vi "RouteExternalInterfaces.vi"(7 "ObjectName":string, 8 "error in (no error)":errorcluster, 9 "ConfigObject":refnum<class "IApplicationConfiguration.lvclass">, 10 "ITAFObject in":refnum<class "ITAFObject.lvclass">, 11 "Variant in":variant) -> (0 "error out":errorcluster, 3 "Variant out":variant)   [LabVIEW 2021, in "Application.lvclass"]
uses:
  Application.lvclass
  Interface_TAF_IApplicationConfiguration/IApplicationConfiguration/IApplicationConfiguration.lvclass
  Interface_TAF_ITAFObject/ITAFObject/ITAFObject.lvclass
  IInterface/IInterface.lvclass
  c3e78f46-7d6b-47a7-82af-8d499459744c.vi
  <vilib>/TriekselSoft/TracerLibrary/TracerLibrary/Tracer/protected/SendMessage.vi
  <vilib>/TriekselSoft/TracerLibrary/TracerLibrary/Tracer/protected/Timestamp.vi
  c3e78f46-7d6b-47a7-82af-8d499459744c.vi/f75db090-0877-4668-94fb-75c2140b1617.vi
  <vilib>/TriekselSoft/TracerLibrary/TracerLibrary/Tracer/Tracer_Level-Debug.vi
  <vilib>/JDP Science/JSONtext/Variant to JSON Text.vi
  <vilib>/TriekselSoft/TracerLibrary/TracerLibrary/Tracer/protected/Tracer_ClassAttributes.vi
  <vilib>/JDP Science/JSONtext/LVClass Serializer/JSONtext LVClass Serializer.lvclass
  Application.lvclass/Application.ctl
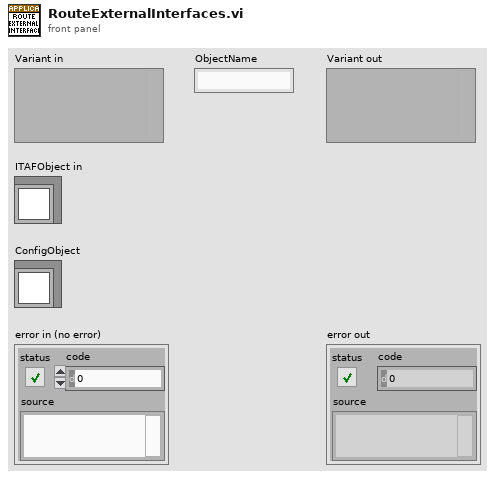
[diagram p1: front panel]
types:
  T1 = typedef "ClusterArrayConversion.lvlib/BundledArray.ctl" = cluster{"Label":string, "Object":refnum<class>, "Array":bool}
  T2 = cluster{"ObjectName":string, "Label":string, "error out":errorcluster}
  T3 = cluster{"ObjectName":string, "Label":string, "ClassName":string}
  T4 = cluster{"ObjectName":string, "Label":string, "class name":string}
  T5 = typedef "IApplicationConfiguration.lvclass/ObjectData.ctl" = cluster{"Label":string, "ObjectName":string, "Type":string}
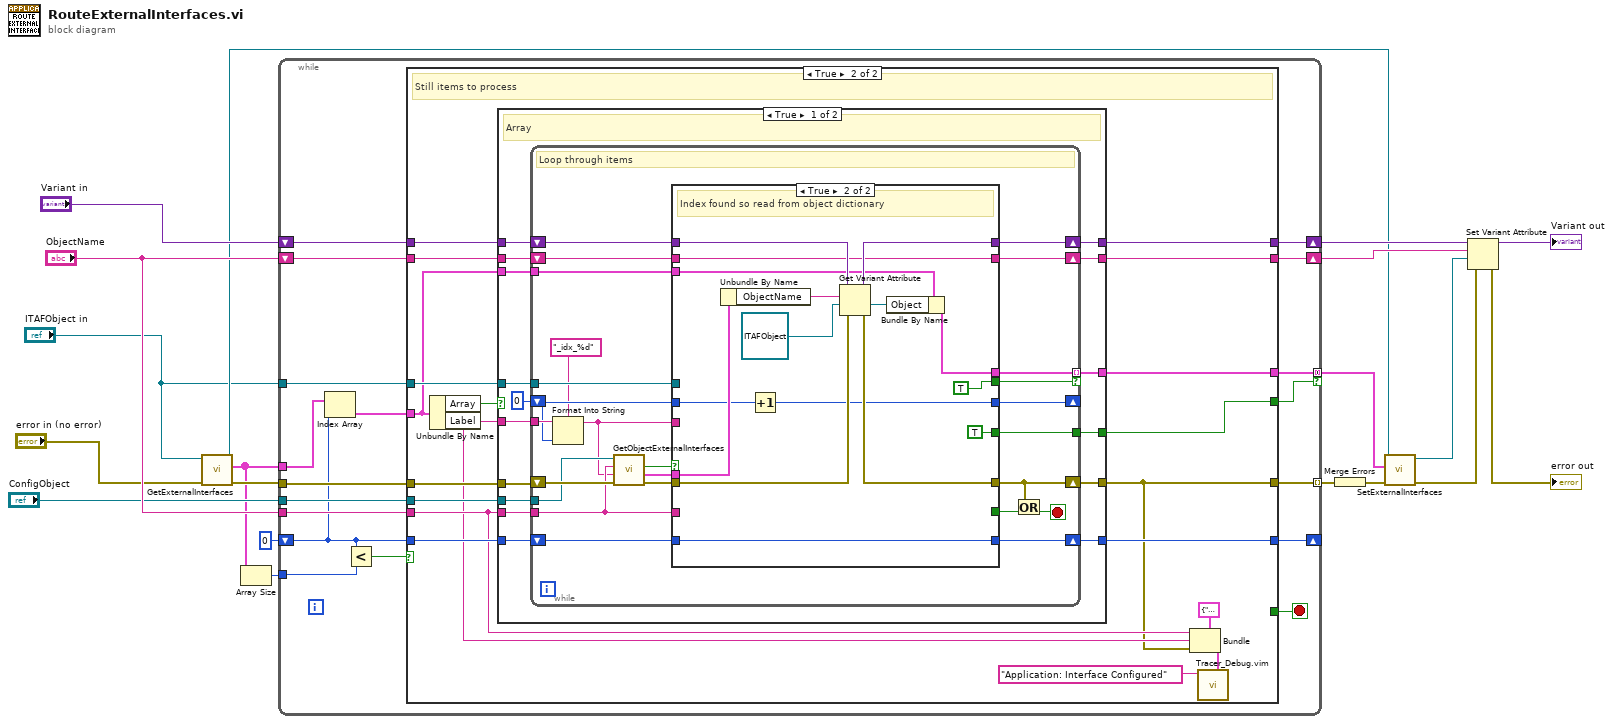
[diagram p0: block diagram]
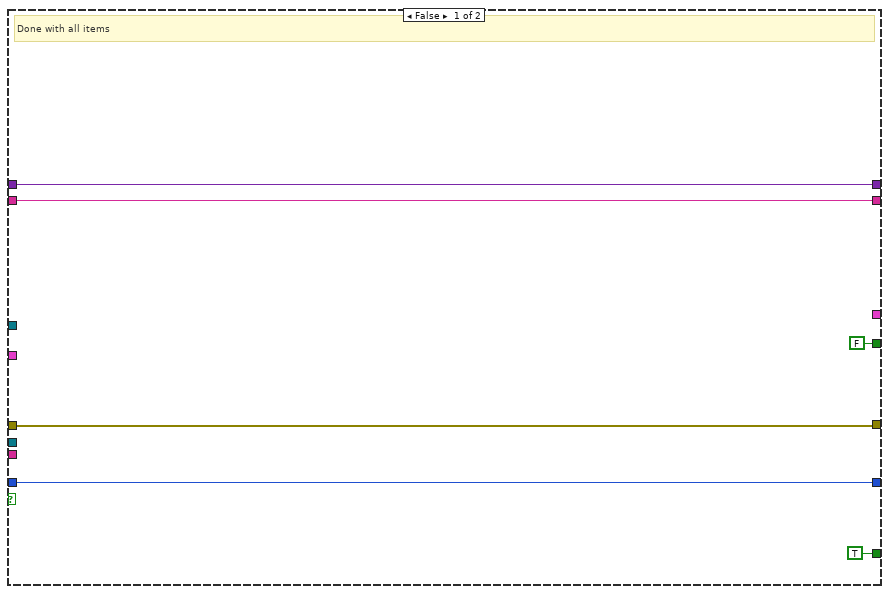
[diagram p2: hidden frame]
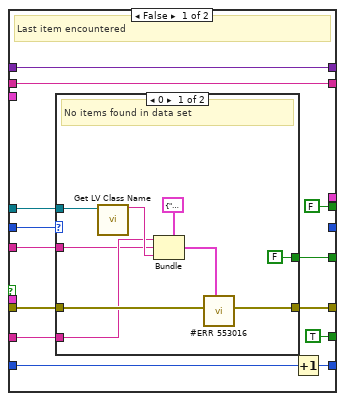
[diagram p3: hidden frame]
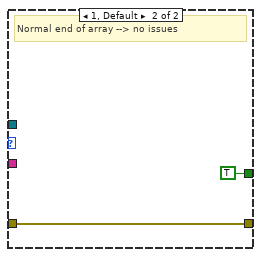
[diagram p4: hidden frame]
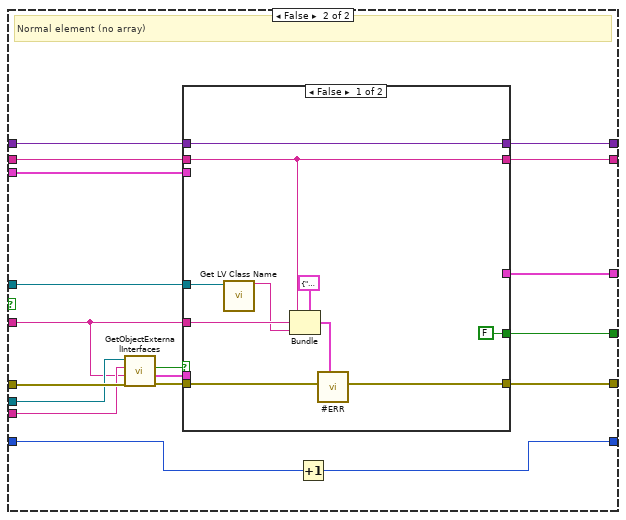
[diagram p5: hidden frame]
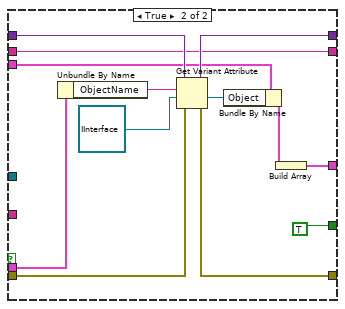
[diagram p6: hidden frame]
diagram:
  n1 = call-dynamic "GetExternalInterfaces.vi"("Error In"="error in (no error)", "object in"="ITAFObject in") -> ("Error Out"=w8:errorcluster, "ExternalInterfaces"=w4:T1[], "object out"=w10:refnum<class "ITAFObject.lvclass">)  [unwired: 7 in]
  n2 = Array Size(array=w4) -> (size(s)=w3:i32)
  n3 = while {
    tunnel: [w37] -> w9 mode=concatenating if=w22
    shift-right: [w33] -> w14
    shift-left: "Variant in" -> [w36]
    shift-right: [w31] -> w15
    shift-left: "ObjectName" -> [w32]
    tunnel: "ConfigObject" -> [w34]
    tunnel: "ObjectName" -> [w30]
    tunnel: w8 -> [w35]
    tunnel: [w29] -> w19 mode=indexing
    tunnel: "ITAFObject in" -> [w28]
    shift-right: [w26] -> _
    shift-left: 0 -> [w25]
    tunnel: w3 -> [w24]
    tunnel: w4 -> [w21]
    stop <- w20 stop-if-true
    n4 = Index Array(array=w21, index=w25) -> (element=w27:T1)
    n5 = Less?(x=w25, y=w24) -> (x < y?=w23:bool)
    n6 = case shown="True" w23 {
      tunnel: [_ w62] -> w37
      tunnel: w36 -> [w43 w61]
      tunnel: w35 -> [w40 w60]
      tunnel: w34 -> [_ w59]
      tunnel: [w43 w58] -> w33
      tunnel: w32 -> [w42 w57]
      tunnel: [w42 w56] -> w31
      tunnel: w30 -> [_ w48]
      tunnel: [w40 w46] -> w29
      tunnel: w28 -> [_ w55]
      tunnel: w27 -> [_ w44]
      tunnel: [w39 w54] -> w26
      tunnel: w25 -> [w39 w53]
      tunnel: [FALSE w45] -> w22
      tunnel: [TRUE _] -> w20
      frame False {
        # "Done with all items"
      }
      frame True {
        # "Still items to process"
        n7 = Unbundle By Name(w44) -> ("Array"=w52:bool, "Label"=w47:string)
        n8 = case shown="True" w52 {
          tunnel: [w78 w161] -> w62
          tunnel: w61 -> [w77 w160]
          tunnel: w60 -> [w76 w159]
          tunnel: w59 -> [w75 w158]
          tunnel: [w74 w155] -> w58
          tunnel: w57 -> [w73 w153]
          tunnel: [w72 w152] -> w56
          tunnel: w48 -> [w71 w151]
          tunnel: [w65 w150] -> w46
          tunnel: w47 -> [w70 w149]
          tunnel: w55 -> [w69 w148]
          tunnel: [w68 w146] -> w54
          tunnel: w53 -> [w67 w147]
          tunnel: [w64 w145] -> w45
          tunnel: w44 -> [w63 w144]
          frame True {
            # "Array"
            n9 = while {
              tunnel: w75 -> [w100]
              tunnel: w71 -> [w84]
              tunnel: w70 -> [w90]
              tunnel: w69 -> [w93]
              shift-right: [w97] -> w74
              shift-left: w77 -> [w102]
              shift-right: [w81] -> w65
              shift-left: w76 -> [w101]
              shift-right: [w94] -> w72
              shift-left: w73 -> [w95]
              shift-right: [w92] -> w68
              shift-left: w67 -> [w91]
              shift-right: [w87] -> _
              shift-left: 0 -> [w89]
              tunnel: [w103] -> w78 mode=indexing if=w86
              tunnel: [w80] -> w64
              tunnel: w63 -> [w79]
              stop <- w82 stop-if-true
              # "Loop through items"
              n10 = Format Into String(format string="_idx_%d", initial string=w90, w89) -> (resulting string=w83:string)  [unwired: 1 in, 1 out]
              n11 = call-dynamic "GetObjectExternalInterfaces.vi"("Error In"=w101, "Label"=w83, "ThisObject"=w84, "object in"=w100) -> ("Error Out"=w98:errorcluster, "ObjectData"=w99:T5, "Valid"=w96:bool)  [unwired: 4 in, 1 out]
              n12 = case shown="True" w96 {
                tunnel: [_ w143] -> w103
                tunnel: w102 -> [w113 w142]
                tunnel: w99 -> [_ w141]
                tunnel: w98 -> [w116 w138]
                tunnel: [w115 w137] -> w81
                tunnel: [w113 w136] -> w97
                tunnel: w84 -> [w114 _]
                tunnel: [w112 w134] -> w94
                tunnel: w95 -> [w112 w134]
                tunnel: w83 -> [w111 _]
                tunnel: w93 -> [w110 _]
                tunnel: w91 -> [w106 w133]
                tunnel: [w107 w133] -> w92
                tunnel: w89 -> [w109 w132]
                tunnel: [_ w131] -> w87
                tunnel: [FALSE TRUE] -> w86
                tunnel: [TRUE _] -> w85
                tunnel: [w104 TRUE] -> w80
                tunnel: w79 -> [_ w128]
                frame False {
                  # "Last item encountered"
                  n13 = case shown="0" w109 {
                    tunnel: w116 -> [w125 w127]
                    tunnel: [w124 w127] -> w115
                    tunnel: w114 -> [w118 _]
                    tunnel: w111 -> [w117 _]
                    tunnel: w110 -> [w123 _]
                    tunnel: [FALSE TRUE] -> w104
                    frame 0 {
                      # "No items found in data set"
                      n14 = call <vilib>:"Get LV Class Name.vi"("object"=w123) -> ("class name"=w122:string)  [unwired: 9 in, 1 out]
                      n15 = Bundle(cluster=T3 {"ObjectName"="", "Label"="", "ClassName"=""}, "ObjectName"=w118, "Label"=w117, "ClassName"=w122) -> (w120:T3)
                      n16 = call "#ERR 553016"("Data"=w120, "error in (no error)"=w125) -> ("error out"=w124:errorcluster)  [unwired: 9 in]
                    }
                    frame 1, Default {
                      # "Normal end of array --> no issues"
                    }
                  }
                  n17 = Increment(x=w106) -> (x+1=w107:i32)
                }
                frame True {
                  # "Index found so read from object dictionary"
                  n18 = Unbundle By Name(w141) -> ("ObjectName"=w140:string)
                  n19 = Increment(x=w132) -> (x+1=w131:i32)
                  n20 = Get Variant Attribute(Variant=w142, name=w140, default value (empty Variant)=refnum<class "ITAFObject.lvclass"> refnum ("NamedCreator"), error in=w138) -> (duplicate Variant=w136:variant, value=w135:refnum<class "ITAFObject.lvclass">, error out=w137:errorcluster)  [unwired: 1 out]
                  n21 = Bundle By Name(cluster=w128, "Object"=w135) -> (w143:T1)
                }
              }
              n22 = Or(x=w81, y=w85) -> (x .or. y?=w82:bool)
            }
          }
          frame False {
            # "Normal element (no array)"
            n23 = call-dynamic "GetObjectExternalInterfaces.vi"("Error In"=w159, "Label"=w149, "ThisObject"=w151, "object in"=w158) -> ("Error Out"=w156:errorcluster, "ObjectData"=w157:T5, "Valid"=w154:bool)  [unwired: 4 in, 1 out]
            n24 = case shown="False" w154 {
              tunnel: [_ w174] -> w161
              tunnel: w160 -> [w168 w183]
              tunnel: w157 -> [_ w182]
              tunnel: w156 -> [w171 w179]
              tunnel: [w170 w178] -> w150
              tunnel: [w168 w177] -> w155
              tunnel: [w163 w175] -> w152
              tunnel: w153 -> [w163 w175]
              tunnel: w149 -> [w167 _]
              tunnel: w148 -> [w166 _]
              tunnel: [FALSE TRUE] -> w145
              tunnel: w144 -> [_ w172]
              frame False {
                n25 = call <vilib>:"Get LV Class Name.vi"("object"=w166) -> ("class name"=w165:string)  [unwired: 9 in, 1 out]
                n26 = Bundle(cluster=T4 {"ObjectName"="", "Label"="", "class name"=""}, "ObjectName"=w163, "Label"=w167, "class name"=w165) -> (w169:T4)
                n27 = call "#ERR"("Data"=w169, "error in (no error)"=w171) -> ("error out"=w170:errorcluster)  [unwired: 9 in]
              }
              frame True {
                n28 = Unbundle By Name(w182) -> ("ObjectName"=w181:string)
                n29 = Get Variant Attribute(Variant=w183, name=w181, default value (empty Variant)=refnum<class "IInterface.lvclass"> refnum ("IInterface"), error in=w179) -> (duplicate Variant=w177:variant, value=w176:refnum<class "IInterface.lvclass">, error out=w178:errorcluster)  [unwired: 1 out]
                n30 = Bundle By Name(cluster=w172, "Object"=w176) -> (w184:T1)
                n31 = Build Array(w184) -> (w174:T1[])
              }
            }
            n32 = Increment(x=w147) -> (x+1=w146:i32)
          }
        }
        n33 = Bundle(cluster=T2 {"ObjectName"="", "Label"="", "error out"={"status"=FALSE, "code"=0, "source"=""}}, "ObjectName"=w48, "Label"=w47, "error out"=w46) -> (w51:T2)
        n34 = call "Tracer_Debug.vim"("Data"=w51, "Text"="Application: Interface Configured") -> ()  [unwired: 9 in, 1 out]
      }
    }
  }
  n35 = Merge Errors(w19) -> (w18:errorcluster)
  n36 = call-dynamic "SetExternalInterfaces.vi"("Error In"=w18, "ExternalInterfaces"=w9, "object in"=w10) -> ("Error Out"=w12:errorcluster, "object out"=w11:refnum<class "ITAFObject.lvclass">)  [unwired: 7 in]
  n37 = Set Variant Attribute(Variant=w14, name=w15, value=w11, error in=w12) -> (Variant out=→"Variant out":variant, error out=→"error out":errorcluster)  [unwired: 1 out]
